vi "Serial_Read.vi"(6 "Task":enum16{"Instant", "All"}(ring), 8 "error in (no error)":errorcluster, 11 "Python":T1) -> (0 "error out":errorcluster, 1 "Text read":string)   [LabVIEW 2020]
uses:
  PythonCtrl.ctl
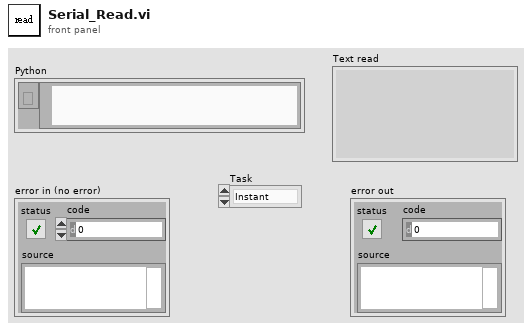
[diagram p1: front panel]
types:
  T1 = typedef "PythonCtrl.ctl" = cluster{"session":refnum<k35>, "PyPath":path}
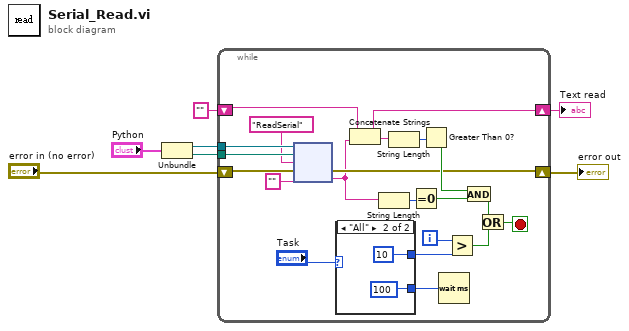
[diagram p0: block diagram]
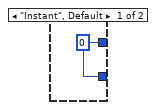
[diagram p2: hidden frame]
diagram:
  n1 = Unbundle("Python") -> ("session"=w6:refnum<k35>, "PyPath"=w5:path)
  n2 = while {
    shift-right: [w10] -> w3
    shift-left: "error in (no error)" -> [w11]
    shift-right: [w24] -> w1
    shift-left: "" -> [w27]
    tunnel: w6 -> [w15]
    tunnel: w5 -> [w14]
    i -> [w19]
    stop <- w21 stop-if-true
    n3 = node(w15, w14, "ReadSerial" ("function name"), w11, "" ("function name")) -> (w10:errorcluster, w9:string)  [unwired: 3 out]
    n4 = case shown="\"All\"" "Task" {
      tunnel: [w28 10 ("y")] -> w18
      tunnel: [w28 u32 100 ("milliseconds to wait")] -> w16
      frame "Instant", Default {
        w28 = 0 ("y")
      }
      frame "All" {
      }
    }
    n5 = Concatenate Strings(w27, w9) -> (w24:string)
    n6 = String Length(string=w9) -> (length=w26:i32)
    n7 = String Length(string=w24) -> (length=w25:i32)
    n8 = Equal To 0?(x=w26) -> (x = 0?=w22:bool)
    n9 = Greater Than 0?(x=w25) -> (x > 0?=w23:bool)
    n10 = Wait (ms)(milliseconds to wait=w16) -> ()  [unwired: 1 out]
    n11 = Greater?(x=w19, y=w18) -> (0:w17:bool)
    n12 = And(x=w23, y=w22) -> (x .and. y?=w20:bool)
    n13 = Or(x=w20, y=w17) -> (x .or. y?=w21:bool)
  }
  "error out" <- w3
  "Text read" <- w1
